vi "校准对话框.vi"(8 "error in":errorcluster {"code" format="%.0x"}, 11 "RS网分地址":refnum<visa-resource-name>="TCPIP0::169.254.134.78::inst0::INSTR") -> (0 "error out":errorcluster {"code" format="%.0x"}, 3 "VISA resource name out":refnum<visa-resource-name>)   [LabVIEW 2015, in "RS.lvclass"]
uses:
  RS.lvclass
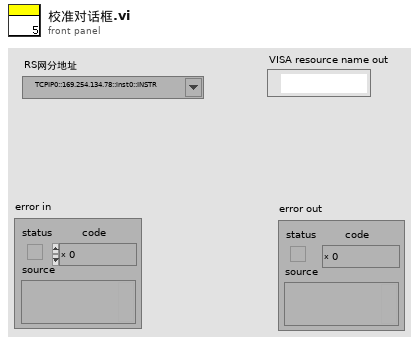
[diagram p1: front panel]
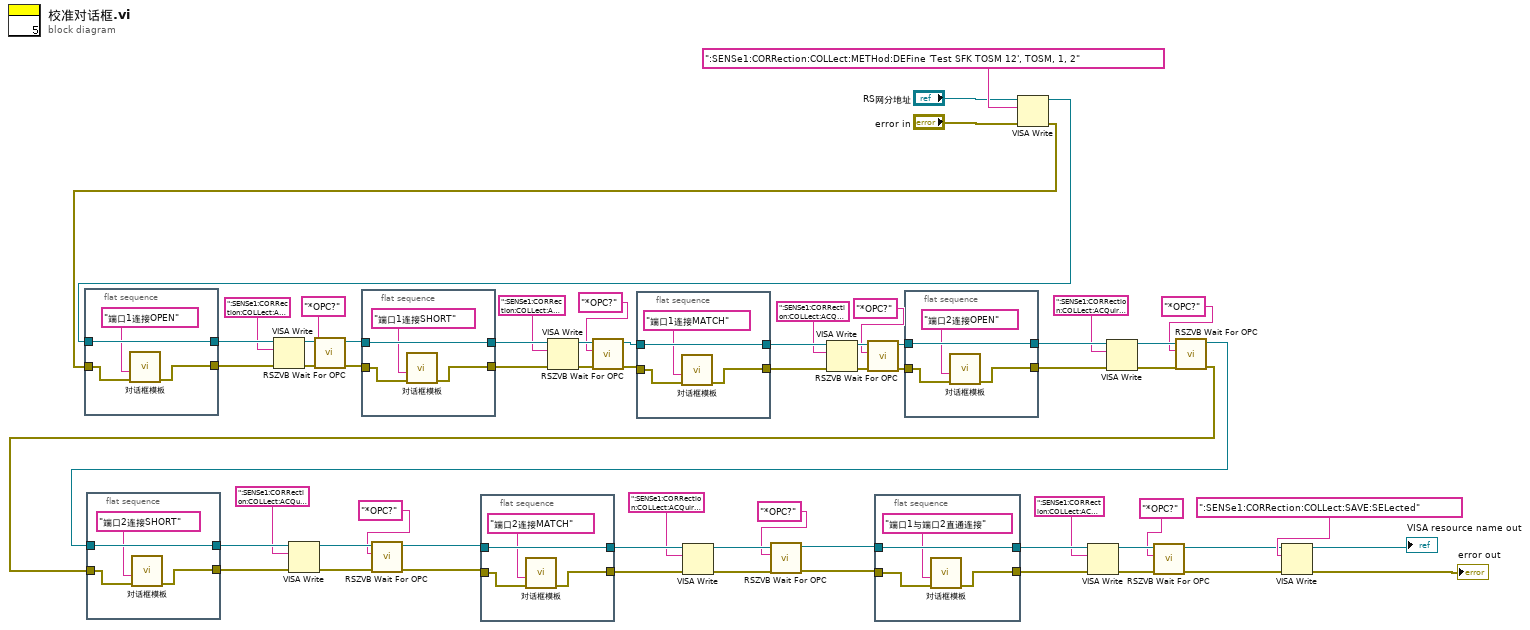
[diagram p0: block diagram]
diagram:
  n1 = flat-sequence {
    tunnel: w4 -> [w67]
    tunnel: w5 -> [w68]
    tunnel: [w66] -> w63
    tunnel: [w68] -> w62
    frame #0 {
      n2 = call "对话框模板.vi"("error in (no error)"=w67, "message"="端口1连接OPEN") -> ("error out"=w66:errorcluster)  [unwired: 8 in, 1 out]
    }
  }
  n3 = flat-sequence {
    tunnel: w22 -> [w71]
    tunnel: w23 -> [w72]
    tunnel: [w70] -> w49
    tunnel: [w72] -> w48
    frame #0 {
      n4 = call "对话框模板.vi"("error in (no error)"=w71, "message"="端口2连接SHORT") -> ("error out"=w70:errorcluster)  [unwired: 8 in, 1 out]
    }
  }
  n5 = VISA Write(VISA resource name=w62, write buffer=":SENSe1:CORRection:COLLect:ACQuire:SELected OPEN, 1", error in (no error)=w63) -> (VISA resource name out=w41:refnum<visa-resource-name>, error out=w40:errorcluster)  [unwired: 1 out]
  n6 = VISA Write(VISA resource name=w48, write buffer=":SENSe1:CORRection:COLLect:ACQuire:SELected SHORT, 2", error in (no error)=w49) -> (VISA resource name out=w21:refnum<visa-resource-name>, error out=w19:errorcluster)  [unwired: 1 out]
  n7 = call "RSZVB Wait For OPC.vi"("error in (no error)"=w40, "Command"="*OPC?", "VISA session"=w41) -> ("error out"=w38:errorcluster, "dup VISA session"=w39:refnum<visa-resource-name>)  [unwired: 6 in, 1 out]
  n8 = flat-sequence {
    tunnel: w38 -> [w75]
    tunnel: w39 -> [w76]
    tunnel: [w74] -> w59
    tunnel: [w76] -> w60
    frame #0 {
      n9 = call "对话框模板.vi"("error in (no error)"=w75, "message"="端口1连接SHORT") -> ("error out"=w74:errorcluster)  [unwired: 8 in, 1 out]
    }
  }
  n10 = call "RSZVB Wait For OPC.vi"("error in (no error)"=w19, "Command"="*OPC?", "VISA session"=w21) -> ("error out"=w17:errorcluster, "dup VISA session"=w18:refnum<visa-resource-name>)  [unwired: 6 in, 1 out]
  n11 = flat-sequence {
    tunnel: w17 -> [w79]
    tunnel: w18 -> [w80]
    tunnel: [w78] -> w50
    tunnel: [w80] -> w51
    frame #0 {
      n12 = call "对话框模板.vi"("error in (no error)"=w79, "message"="端口2连接MATCH") -> ("error out"=w78:errorcluster)  [unwired: 8 in, 1 out]
    }
  }
  n13 = VISA Write(VISA resource name=w60, write buffer=":SENSe1:CORRection:COLLect:ACQuire:SELected SHORT, 1", error in (no error)=w59) -> (VISA resource name out=w36:refnum<visa-resource-name>, error out=w35:errorcluster)  [unwired: 1 out]
  n14 = call "RSZVB Wait For OPC.vi"("error in (no error)"=w35, "Command"="*OPC?", "VISA session"=w36) -> ("error out"=w33:errorcluster, "dup VISA session"=w34:refnum<visa-resource-name>)  [unwired: 6 in, 1 out]
  n15 = flat-sequence {
    tunnel: w33 -> [w83]
    tunnel: w34 -> [w84]
    tunnel: [w82] -> w57
    tunnel: [w84] -> w56
    frame #0 {
      n16 = call "对话框模板.vi"("error in (no error)"=w83, "message"="端口1连接MATCH") -> ("error out"=w82:errorcluster)  [unwired: 8 in, 1 out]
    }
  }
  n17 = VISA Write(VISA resource name=w51, write buffer=":SENSe1:CORRection:COLLect:ACQuire:SELected MATCH, 2", error in (no error)=w50) -> (VISA resource name out=w16:refnum<visa-resource-name>, error out=w14:errorcluster)  [unwired: 1 out]
  n18 = call "RSZVB Wait For OPC.vi"("error in (no error)"=w14, "Command"="*OPC?", "VISA session"=w16) -> ("error out"=w13:errorcluster, "dup VISA session"=w15:refnum<visa-resource-name>)  [unwired: 6 in, 1 out]
  n19 = VISA Write(VISA resource name=w56, write buffer=":SENSe1:CORRection:COLLect:ACQuire:SELected MATCH, 1", error in (no error)=w57) -> (VISA resource name out=w31:refnum<visa-resource-name>, error out=w30:errorcluster)  [unwired: 1 out]
  n20 = call "RSZVB Wait For OPC.vi"("error in (no error)"=w30, "Command"="*OPC?", "VISA session"=w31) -> ("error out"=w28:errorcluster, "dup VISA session"=w29:refnum<visa-resource-name>)  [unwired: 6 in, 1 out]
  n21 = flat-sequence {
    tunnel: w13 -> [w87]
    tunnel: w15 -> [w88]
    tunnel: [w86] -> w45
    tunnel: [w88] -> w44
    frame #0 {
      n22 = call "对话框模板.vi"("error in (no error)"=w87, "message"="端口1与端口2直通连接") -> ("error out"=w86:errorcluster)  [unwired: 8 in, 1 out]
    }
  }
  n23 = flat-sequence {
    tunnel: w28 -> [w91]
    tunnel: w29 -> [w92]
    tunnel: [w90] -> w53
    tunnel: [w92] -> w54
    frame #0 {
      n24 = call "对话框模板.vi"("error in (no error)"=w91, "message"="端口2连接OPEN") -> ("error out"=w90:errorcluster)  [unwired: 8 in, 1 out]
    }
  }
  n25 = VISA Write(VISA resource name="RS网分地址", write buffer=":SENSe1:CORRection:COLLect:METHod:DEFine 'Test SFK TOSM 12', TOSM, 1, 2", error in (no error)="error in") -> (VISA resource name out=w5:refnum<visa-resource-name>, error out=w4:errorcluster)  [unwired: 1 out]
  n26 = VISA Write(VISA resource name=w44, write buffer=":SENSe1:CORRection:COLLect:ACQuire:SELected THROUGH, 1, 2", error in (no error)=w45) -> (VISA resource name out=w11:refnum<visa-resource-name>, error out=w9:errorcluster)  [unwired: 1 out]
  n27 = VISA Write(VISA resource name=w54, write buffer=":SENSe1:CORRection:COLLect:ACQuire:SELected OPEN, 2", error in (no error)=w53) -> (VISA resource name out=w26:refnum<visa-resource-name>, error out=w25:errorcluster)  [unwired: 1 out]
  n28 = call "RSZVB Wait For OPC.vi"("error in (no error)"=w9, "Command"="*OPC?", "VISA session"=w11) -> ("error out"=w8:errorcluster, "dup VISA session"=w10:refnum<visa-resource-name>)  [unwired: 6 in, 1 out]
  n29 = call "RSZVB Wait For OPC.vi"("error in (no error)"=w25, "Command"="*OPC?", "VISA session"=w26) -> ("error out"=w22:errorcluster, "dup VISA session"=w23:refnum<visa-resource-name>)  [unwired: 6 in, 1 out]
  n30 = VISA Write(VISA resource name=w10, write buffer=":SENSe1:CORRection:COLLect:SAVE:SELected", error in (no error)=w8) -> (VISA resource name out=→"VISA resource name out":refnum<visa-resource-name>, error out=→"error out":errorcluster)  [unwired: 1 out]
